vi "Fast_string_Replace.vi"(3 "Replace match with:":string, 4 "Input String":string, 5 "regular expression":string) -> (0 "Number Found":i32, 1 "Output String":string)   [LabVIEW 2010]
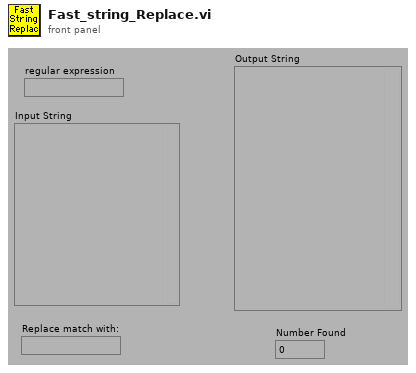
[diagram p1: front panel]
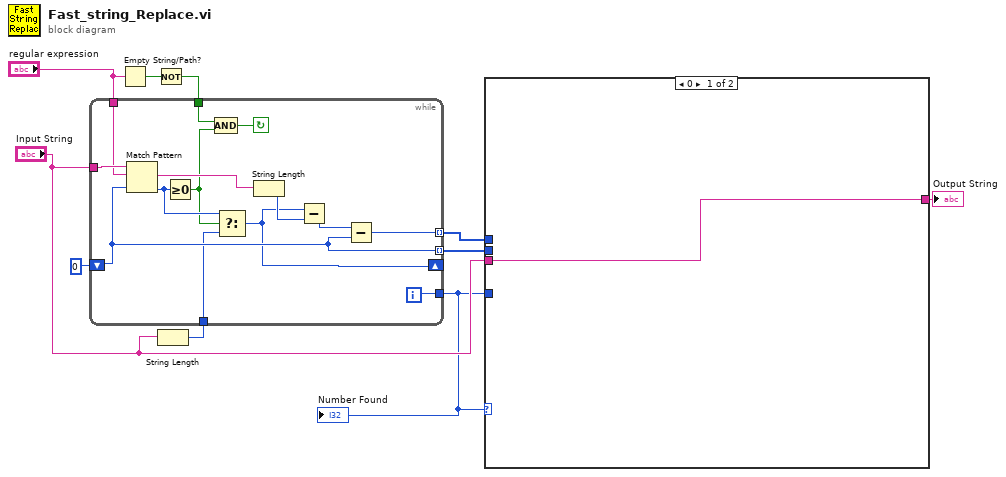
[diagram p0: block diagram]
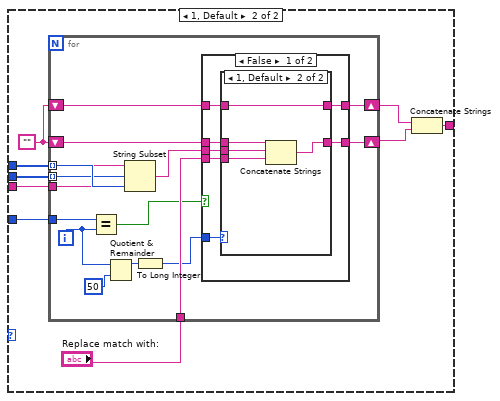
[diagram p2: hidden frame]
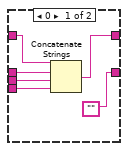
[diagram p3: hidden frame]
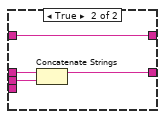
[diagram p4: hidden frame]
diagram:
  n1 = Empty String/Path?(string/path="regular expression") -> (empty?=w2:bool)
  n2 = Not(x=w2) -> (.not. x?=w1:bool)
  n3 = String Length(string="Input String") -> (length=w6:i32)
  n4 = while {
    tunnel: w1 -> [w12]
    tunnel: [w14] -> w4
    tunnel: w6 -> [w16]
    tunnel: "regular expression" -> [w18]
    tunnel: [w19] -> w8 mode=indexing
    tunnel: [w20] -> w9 mode=indexing
    tunnel: "Input String" -> [w23]
    shift-left: 0 -> [w19]
    shift-right: [w15] -> _
    i -> [w14]
    stop <- w11 continue-if-true
    n5 = Match Pattern(string=w23, regular expression=w18, offset (0)=w19) -> (match substring=w24:string, offset past match=w17:i32)  [unwired: 2 out]
    n6 = Greater Or Equal To 0?(x=w17) -> (x >= 0?=w13:bool)
    n7 = Compound Arithmetic op=AND(w12, w13) -> (w11:bool)
    n8 = Select(t=w17, s=w13, f=w16) -> (s? t:f=w15:i32)
    n9 = String Length(string=w24) -> (length=w22:i32)
    n10 = Subtract(x=w15, y=w22) -> (x-y=w21:i32)
    n11 = Subtract(x=w21, y=w19) -> (x-y=w20:i32)
  }
  "Number Found" <- w4
  n12 = case shown="0" w4 {
    tunnel: w9 -> [_ w33]
    tunnel: w8 -> [_ w32]
    tunnel: "Input String" -> [w25 w31]
    tunnel: w4 -> [_ w30]
    tunnel: [w25 w26] -> w5
    frame 0 {
    }
    frame 1, Default {
      w29 = ""
      n13 = for {
        shift-right: [w43] -> w27
        shift-left: w29 -> [w49]
        tunnel: "Replace match with:" -> [w48]
        tunnel: w33 -> [w47] mode=indexing
        tunnel: w32 -> [w46] mode=indexing
        tunnel: w31 -> [w45]
        tunnel: w30 -> [w42]
        shift-right: [w35] -> w28
        shift-left: w29 -> [w36]
        i -> [w38]
        n14 = Equal?(x=w42, y=w38) -> (x = y?=w41:bool)
        n15 = Quotient & Remainder(x=w38, y=50) -> (x-y*floor(x/y)=w40:i32)  [unwired: 1 out]
        n16 = String Subset(string=w45, offset (0)=w46, length (rest)=w47) -> (substring=w44:string)
        n17 = To Long Integer(number=w40) -> (32bit integer=w37:i32)
        n18 = case shown="False" w41 {
          tunnel: w49 -> [w56 w71]
          tunnel: w48 -> [w55 _]
          tunnel: w44 -> [w54 w70]
          tunnel: [w53 w69] -> w43
          tunnel: w37 -> [w52 _]
          tunnel: w36 -> [w51 w68]
          tunnel: [w50 w68] -> w35
          frame False {
            n19 = case shown="1, Default" w52 {
              tunnel: w56 -> [w62 w66]
              tunnel: w55 -> [w61 w64]
              tunnel: w54 -> [w60 w65]
              tunnel: ["" w63] -> w53
              tunnel: w51 -> [w59 w67]
              tunnel: [w58 w67] -> w50
              frame 0 {
                n20 = Concatenate Strings(w59, w62, w60, w61) -> (w58:string)
              }
              frame 1, Default {
                n21 = Concatenate Strings(w66, w65, w64) -> (w63:string)
              }
            }
          }
          frame True {
            n22 = Concatenate Strings(w71, w70) -> (w69:string)
          }
        }
      }
      n23 = Concatenate Strings(w28, w27) -> (w26:string)
    }
  }
  "Output String" <- w5
